vi "Resolve Waits.vi"(9 "New Map in":refnum<class "Map.lvclass">, 11 "Map in":refnum<class "Map.lvclass">) -> (1 "New Map out":refnum<class "Map.lvclass">)   [LabVIEW 2020]
uses:
  Map.lvclass
  Map.lvclass/Map.ctl
  Action.ctl
  SquareBattle.lvlib
  Square/Square.lvclass
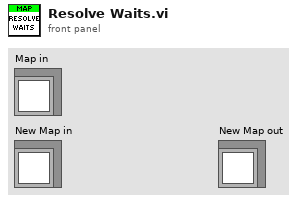
[diagram p1: front panel]
types:
  T1 = typedef "SquareBattle.lvlib/Action.ctl" = enum16{"Wait", "Move", "Attack", "Replicate"}
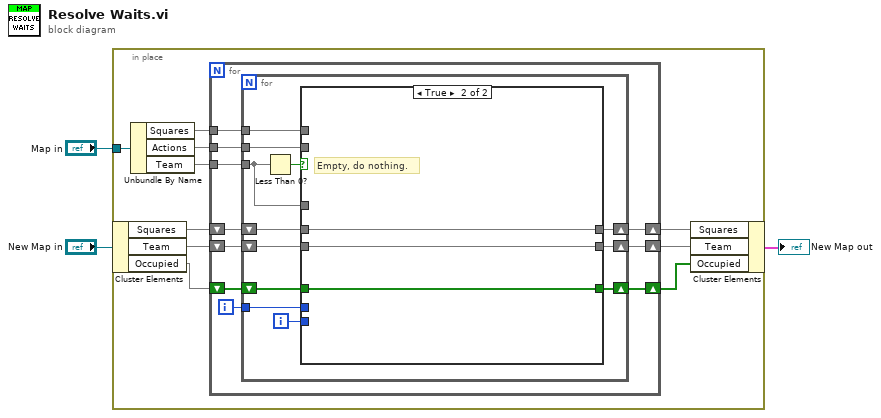
[diagram p0: block diagram]
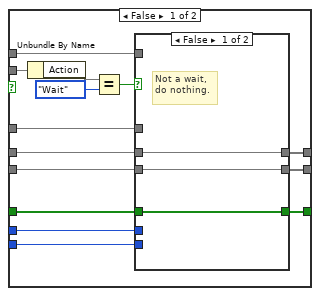
[diagram p2: hidden frame]
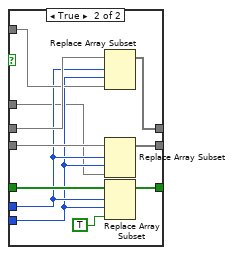
[diagram p3: hidden frame]
diagram:
  n1 = in-place {
    in-place-border: "Map in" -> [w12]
    n2 = in-place-cluster #1("New Map in") -> ("Squares"=w13, "Team"=w9, "Occupied"=w5)
    n3 = Unbundle By Name(w12) -> ("Squares"=w11, "Actions"=w10, "Team"=w6)
    n4 = for {
      shift-right: [w21] -> w8
      shift-left: w13 -> [w23]
      tunnel: w11 -> [w18]
      tunnel: w10 -> [w19]
      shift-right: [w20] -> w7
      shift-left: w9 -> [w22]
      tunnel: w6 -> [w17]
      shift-right: [w14] -> w4
      shift-left: w5 -> [w15]
      i -> [w16]
      n5 = for {
        shift-right: [w29] -> w21
        shift-left: w23 -> [w33]
        shift-right: [w28] -> w20
        shift-left: w22 -> [w32]
        tunnel: w19 -> [w35]
        tunnel: w18 -> [w27]
        tunnel: w17 -> [w24]
        tunnel: w16 -> [w31]
        shift-right: [w25] -> w14
        shift-left: w15 -> [w26]
        i -> [w30]
        n6 = Less Than 0?(x=w24) -> (x < 0?=w34:bool)
        n7 = case shown="True" w34 {
          tunnel: w35 -> [w49 _]
          tunnel: w33 -> [w45 w66]
          tunnel: w32 -> [w44 w65]
          tunnel: w31 -> [w41 _]
          tunnel: w30 -> [w40 _]
          tunnel: [w43 w66] -> w29
          tunnel: [w42 w65] -> w28
          tunnel: w27 -> [w39 _]
          tunnel: w26 -> [w38 w64]
          tunnel: [w37 w64] -> w25
          tunnel: w24 -> [w36 _]
          frame False {
            n8 = Unbundle By Name(w49) -> ("Action"=w48)
            n9 = Equal?(x=w48, y=Action."Wait") -> (x = y?=w46:bool)
            n10 = case shown="False" w46 {
              tunnel: w45 -> [w52 w63]
              tunnel: w44 -> [w51 w62]
              tunnel: [w52 w59] -> w43
              tunnel: [w51 w61] -> w42
              tunnel: w41 -> [_ w56]
              tunnel: w40 -> [_ w55]
              tunnel: w39 -> [_ w60]
              tunnel: w38 -> [w50 w58]
              tunnel: [w50 w57] -> w37
              tunnel: w36 -> [_ w53]
              frame False {
                # "Not a wait, do nothing."
              }
              frame True {
                n11 = Replace Array Subset(array=w63, new element=w60, index (row)=w56, index (col)=w55) -> (w59:void[])
                n12 = Replace Array Subset(array=w62, new element=w53, index (row)=w56, index (col)=w55) -> (w61:void[])
                n13 = Replace Array Subset(array=w58, new element=TRUE ("new element/subarray"), index (row)=w56, index (col)=w55) -> (w57:bool[])
              }
            }
          }
          frame True {
            # "Empty, do nothing."
          }
        }
      }
    }
    n14 = in-place-cluster #1("Squares"=w8, "Team"=w7, "Occupied"=w4) -> (→"New Map out":cluster{})
  }
